vi "GetBOTToken.vi"(0 "reference in":refnum<class "TelegramBOT.lvclass">, 5 "error in (no error)":errorcluster) -> (14 "reference out":refnum<class "TelegramBOT.lvclass">, 16 "BOTToken":string, 19 "error out":errorcluster)   [LabVIEW 2014, in "TelegramBOT.lvclass"]
uses:
  TelegramBOT.lvclass
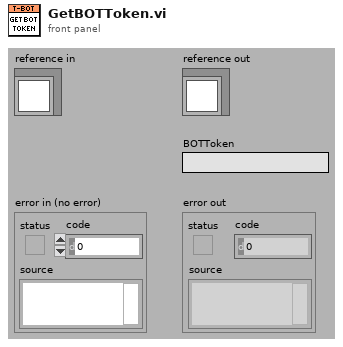
[diagram p1: front panel]
types:
  T1 = typedef "TelegramBOT.lvclass/ObjectAttributes.ctl" = cluster{"BOTToken":string, "AllowedSenders":string[], "AllowedMessages":string[]}
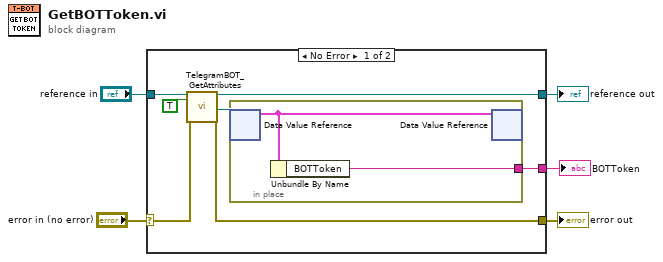
[diagram p0: block diagram]
diagram:
  n1 = case shown="No Error" "error in (no error)" {
    selector: "error in (no error)" -> [w12 w16]
    tunnel: [w11 w16] -> w4
    tunnel: [w9 w15] -> w2
    tunnel: "reference in" -> [w10 w15]
    tunnel: [w6 _] -> w1
    frame No Error {
      n2 = call "TelegramBOT_GetAttributes.vi"("reference in"=w10, "OnlyGetDvrReference(False)"=TRUE, "error in (no error)"=w12) -> ("reference out"=w9:refnum<class "TelegramBOT.lvclass">, "DataRef"=w8:refnum<data-value>, "error out"=w11:errorcluster)  [unwired: 13 in, 1 out]
      n3 = in-place {
        in-place-border: [w14] -> w6
        n4 = in-place-dvr #1(w8) -> (w13:T1)  [unwired: 1 out]
        n5 = Unbundle By Name(w13) -> ("BOTToken"=w14:string)
        n6 = in-place-dvr #1(w13) -> ()  [unwired: 2 out]
      }
    }
    frame Error {
    }
  }
  "error out" <- w4
  "reference out" <- w2
  "BOTToken" <- w1
